vi "c_Send Signal to Acquire Module.vi"() -> (1 "Case Label":T1)   [LabVIEW 2018, in "Aging View.lvclass"]
uses:
  Aging View.lvclass
  <vilib>/addons/_Workers/Library/Case Label.ctl
  <vilib>/addons/_Workers/Library/Workers.lvlib
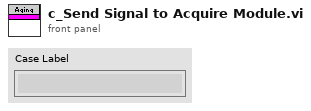
[diagram p1: front panel]
types:
  T1 = typedef "Workers.lvlib/Case Label.ctl" = string
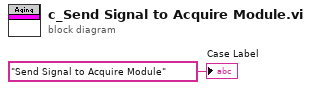
[diagram p0: block diagram]
diagram:
  "Case Label" <- T1 "Send Signal to Acquire Module" ("Case Label")
